vi "Timer_Main_1.vi"() -> ()   [LabVIEW 2020]
uses:
  Door_class/Door.lvclass
panel:
  out "Open?":bool
  in  "Close":bool
  in  "Open":bool
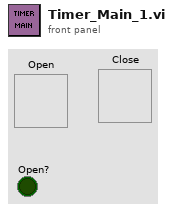
[diagram p1: front panel]
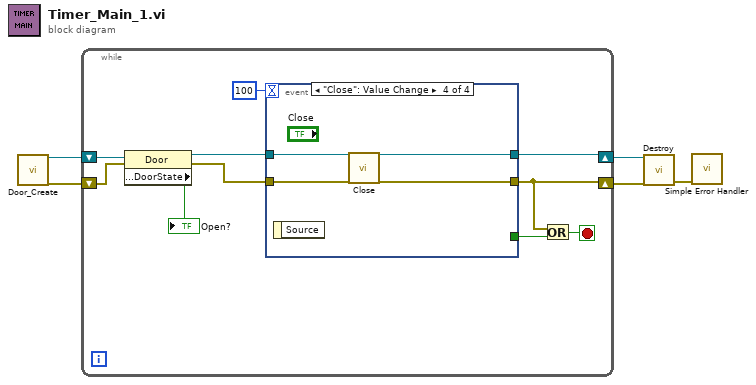
[diagram p0: block diagram]
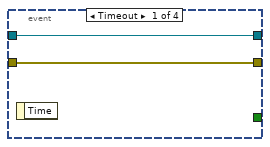
[diagram p2: hidden frame]
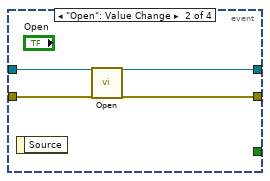
[diagram p3: hidden frame]
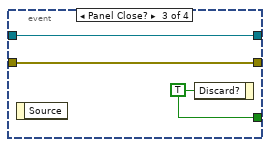
[diagram p4: hidden frame]
diagram:
  n1 = call "Door_Create.vi"() -> ("reference out"=w5:refnum<class "Door.lvclass">, "error out"=w4:errorcluster)  [unwired: 18 in]
  n2 = while {
    shift-right: [w11] -> w3
    shift-left: w5 -> [w14]
    shift-right: [w8] -> w2
    shift-left: w4 -> [w13]
    stop <- w6 stop-if-true
    n3 = property class="Door"(reference=w14, error in=w13) -> (reference out=w12:refnum<class "Door.lvclass">, error out=w10:errorcluster, "properties:DoorState"=→"Open?":bool)
    n4 = event shown="[3] \"Close\": Value Change" {
      selector: _ -> [_ _ _ _]
      dyn-events: _ -> [_ _ _ _]
      timeout: 100 -> [_ _ _ _]
      tunnel: w12 -> [w17 w21 w23 w28]
      tunnel: [w17 w18 w23 w25] -> w11
      tunnel: w10 -> [w16 w20 w24 w27]
      tunnel: [w16 w19 w24 w26] -> w8
      tunnel: [_ _ w22 _] -> w7
      event Timeout {
        n5 = event-data() -> ()  [unwired: 1 in, 1 out]
      }
      event "Open": Value Change {
        n6 = event-data() -> ()  [unwired: 1 in, 1 out]
        n7 = call-dynamic "Open.vi"("reference in"=w21, "error in (no error)"=w20) -> ("reference out"=w18:refnum<class "Door.lvclass">, "error out"=w19:errorcluster)  [unwired: 16 in]
      }
      event Panel Close? {
        w22 = TRUE ("Discard?")
        n8 = event-data() -> ()  [unwired: 1 in, 1 out]
        n9 = event-data("Discard?"=w22) -> ()  [unwired: 1 in, 1 out]
      }
      event "Close": Value Change {
        n10 = event-data() -> ()  [unwired: 1 in, 1 out]
        n11 = call-dynamic "Close.vi"("reference in"=w28, "error in (no error)"=w27) -> ("reference out"=w25:refnum<class "Door.lvclass">, "error out"=w26:errorcluster)  [unwired: 16 in]
      }
    }
    n12 = Or(x=w8, y=w7) -> (x .or. y?=w6:bool)
  }
  n13 = call-dynamic "Destroy.vi"("reference in"=w3, "error in (no error)"=w2) -> ("error out"=w1:errorcluster)  [unwired: 16 in, 1 out]
  n14 = call <vilib>:"Simple Error Handler.vi"("error in (no error)"=w1) -> ()  [unwired: 4 in, 5 out]
